vi "G_Enfriamiento.vi"() -> ()   [LabVIEW 2020]
panel:
  out "Enfriamiento":T1
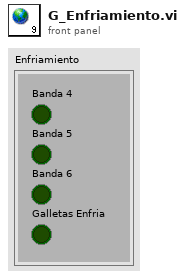
[diagram p1: front panel]
types:
  T1 = cluster{"Banda 4":bool, "Banda 5":bool, "Banda 6":bool, "Galletas Enfria":bool}
diagram:
